vi "Making by Hot.vi"(0 "configuration file path":path caption="配置文件的路径", 1 "making by hot msic inf":T1) -> ()   [LabVIEW 2014]
uses:
  Ctl.xio/Making by Hot msic ctl.ctl
  SubVIS.xio/DataSocket/DataSocket_Tags.ctl
  Ctl.xio/part type.ctl
  SubVIS.xio/Creat Write List VI's/DefCtrl/Station.ctl
  <vilib>/Utility/file.llb/Read From Spreadsheet File (string).vi
panel:
  in  "SQL information":string
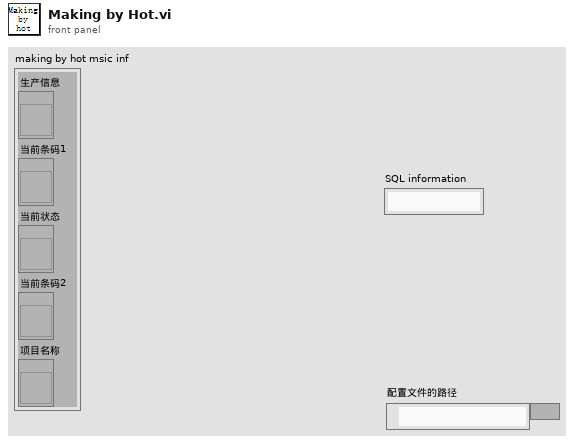
[diagram p1: front panel]
types:
  T1 = cluster{"生产信息":refnum<vi>, "当前条码1":refnum<vi>, "当前状态":refnum<vi>, "当前条码2":refnum<vi>, "项目名称":refnum<vi>}
  T2 = typedef "Station.ctl" = enum16{"粗切工位", "热处理工位", "精切工位", "PDF焊接工位", "打凹点预载力工位", "收卷工位", "EOL工位"}
  T3 = typedef "Making by Hot msic ctl.ctl" = cluster{"configuration file path":path, "DsOut":T4[], "BarCode1":string, "Hopper car information":cluster{"Hopper car code":string, "Hopper car No":string, "plate No":string}, "pallet.produced number":i32, "SQL information":string, "Database":string[], "Serial number":i32, "database path":path, "making by hot msic inf":cluster{"生产信息":refnum<vi>, "当前条码1":refnum<vi>, "当前状态":refnum<vi>, "当前条码2":refnum<vi>, "项目名称":refnum<vi>}, "scnner1 connect id":refnum<k5>, "scnner2 connect id":refnum<k5>, "scanner1 IP":string, "scanner2 IP":string, "BarCode2":string, "Heating process parameters":cluster{"heating start":string, "heating finish":string, "Heating time use":u32}, "part type":T5}
  T4 = typedef "DataSocket_Tags.ctl" = cluster{"Ds ID":refnum<k13>, "Tag":string}
  T5 = typedef "part type.ctl" = cluster{"项目号":string, "物料代码":string, "零件号":string, "供应商编码":string, "产线编码":string, "客户代码":string, "颜色代码":string, "托盘上限":i32, "加热温度":string, "加热时长":string, "EOL Stations":string}
  T6 = cluster{"Hopper car code":string, "Hopper car No":string, "plate No":string}
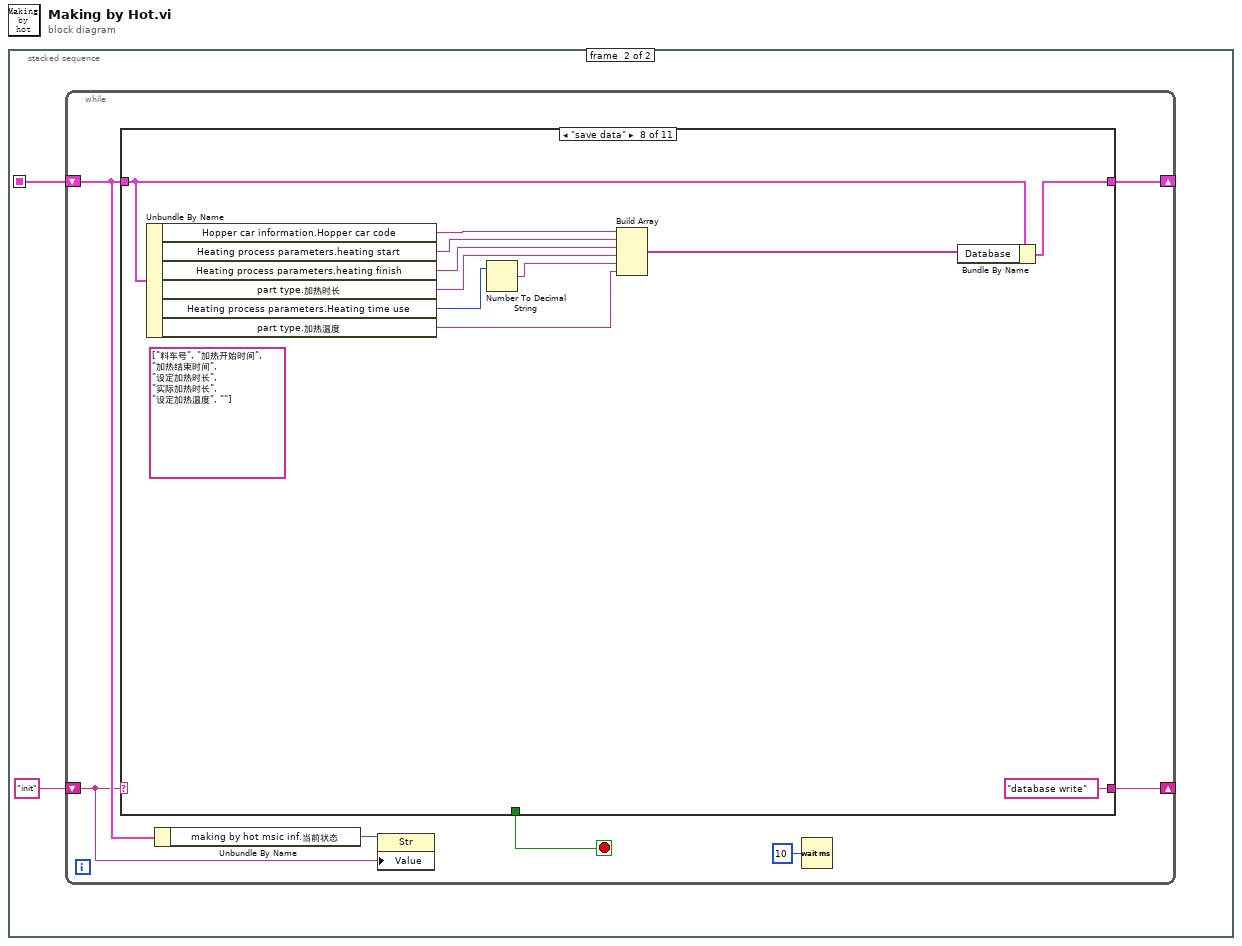
[diagram p0: block diagram]
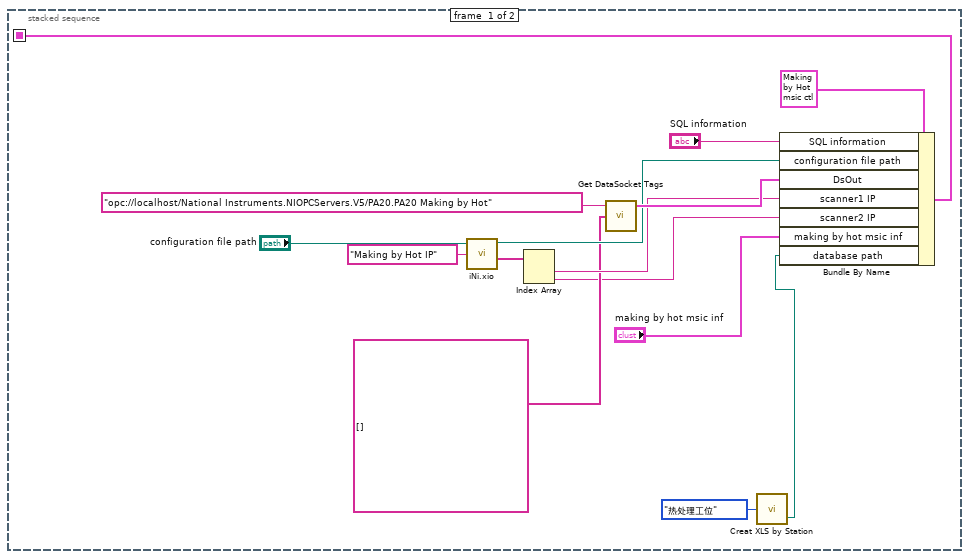
[diagram p2: hidden frame]
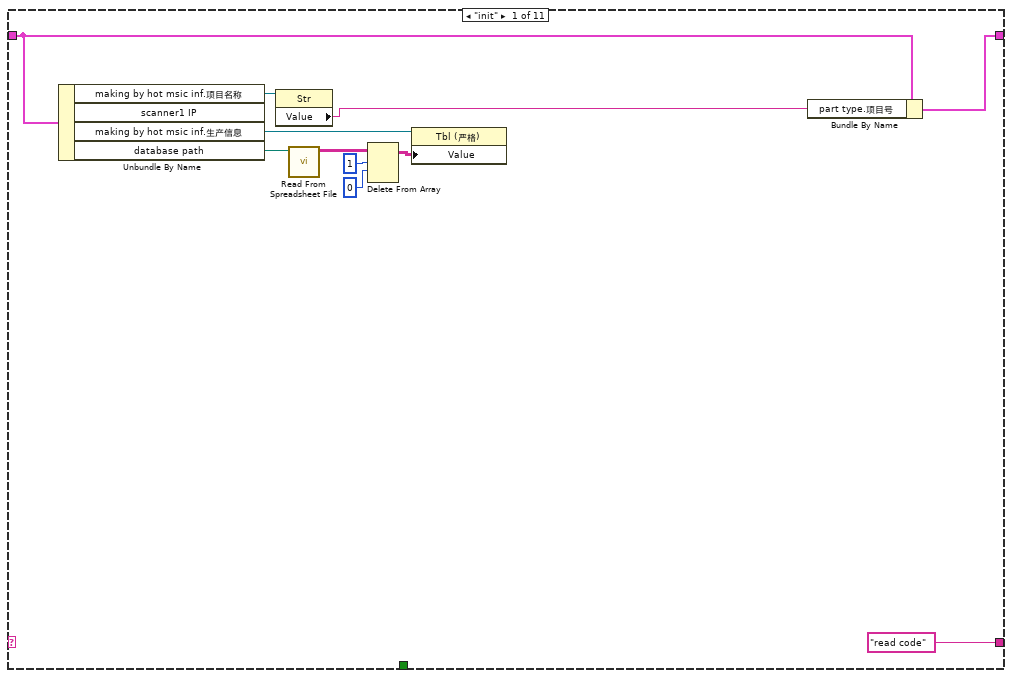
[diagram p3: hidden frame]
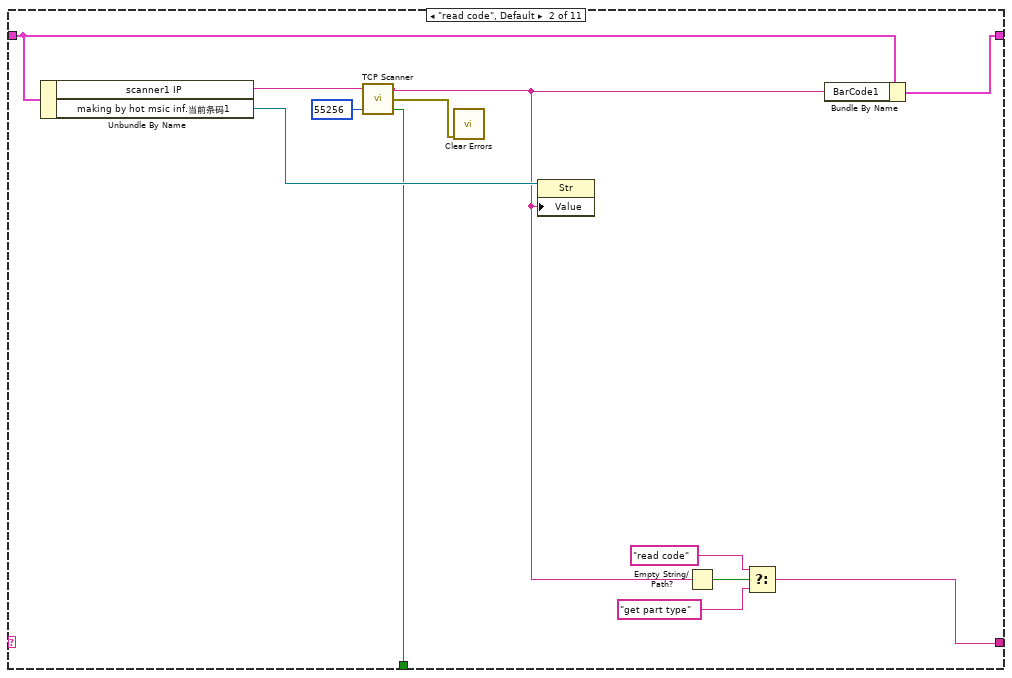
[diagram p4: hidden frame]
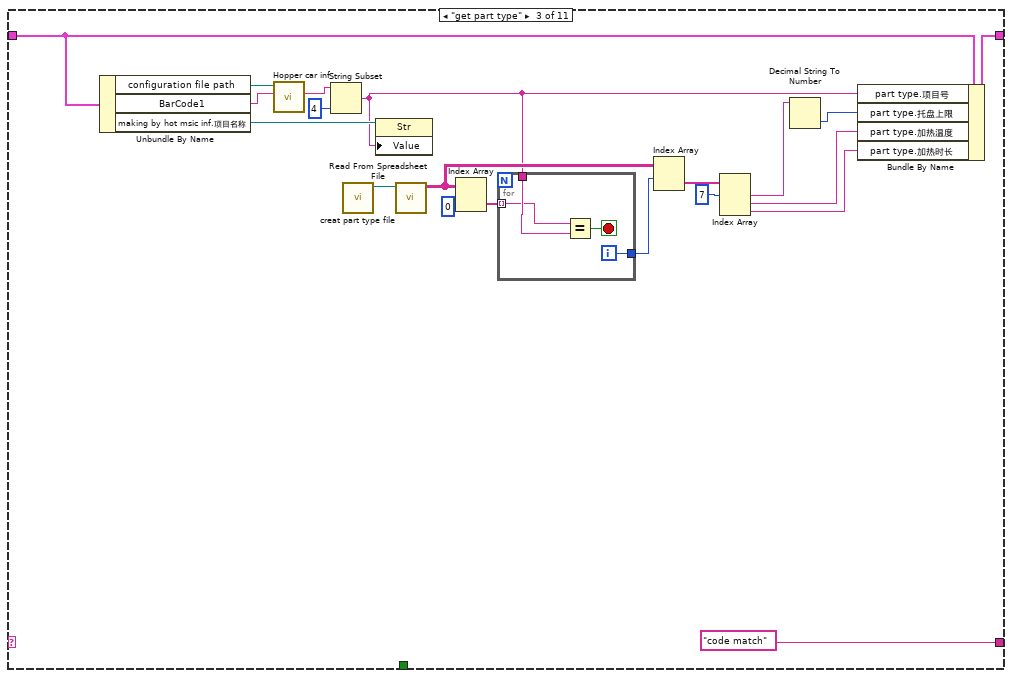
[diagram p5: hidden frame]
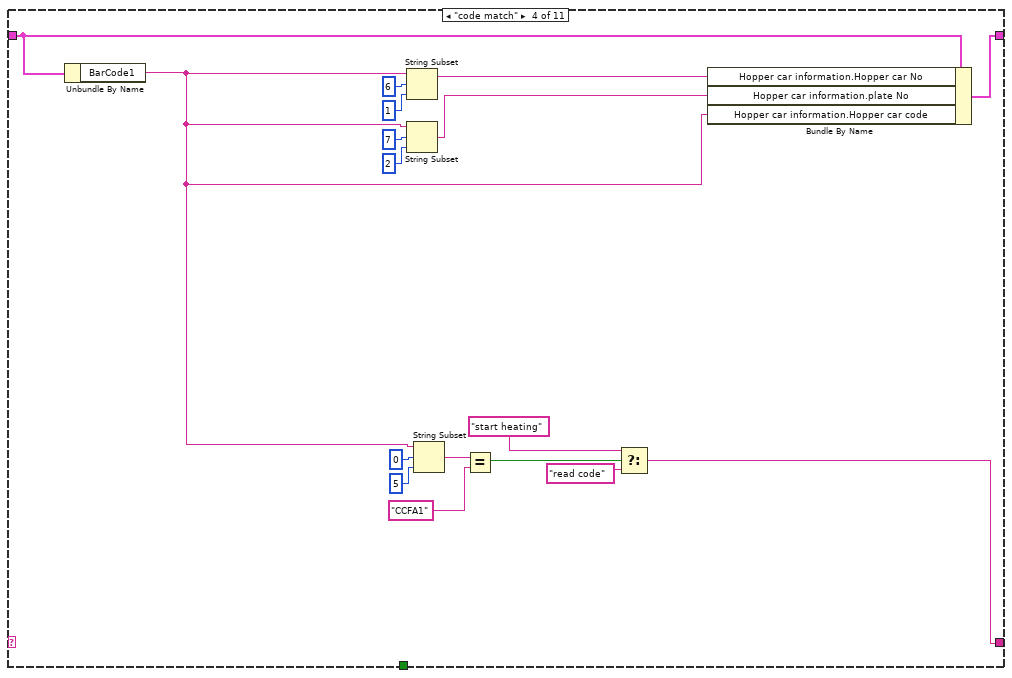
[diagram p6: hidden frame]
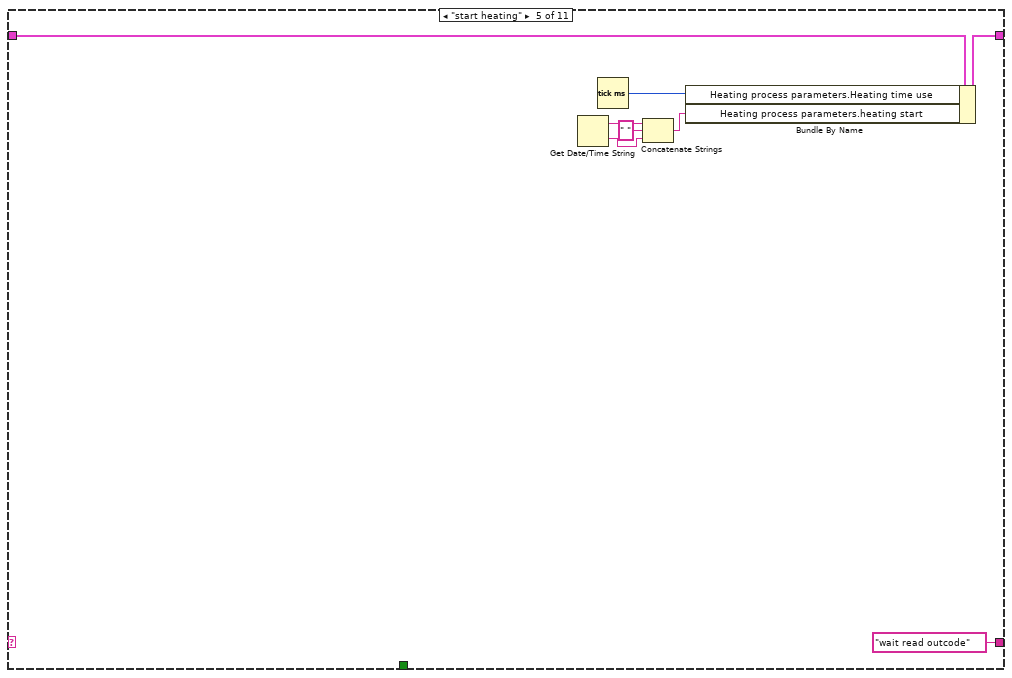
[diagram p7: hidden frame]
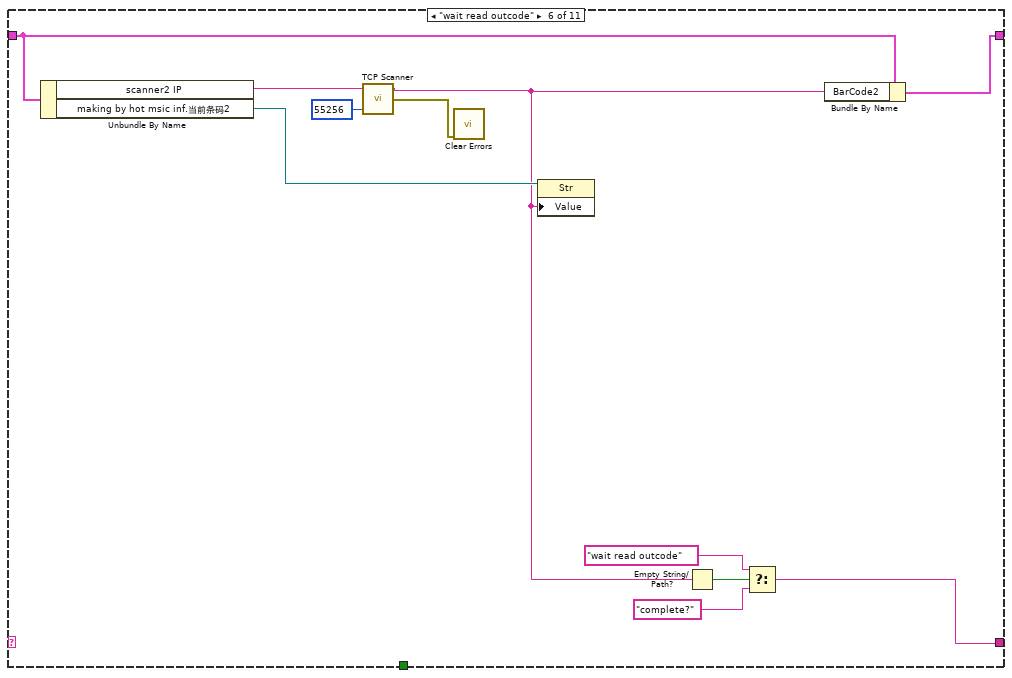
[diagram p8: hidden frame]
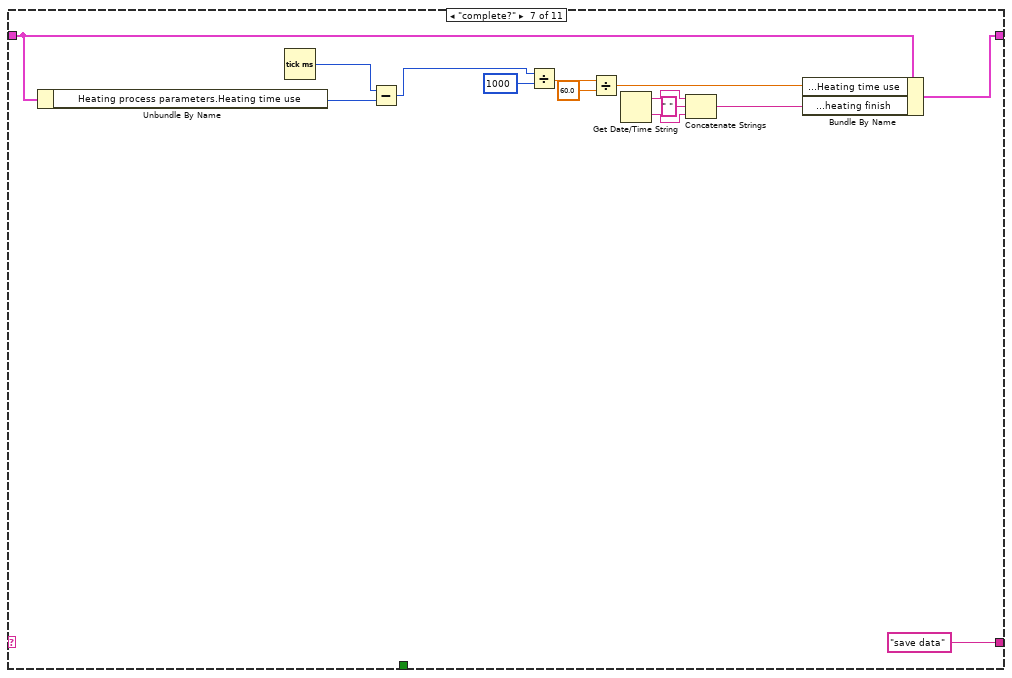
[diagram p9: hidden frame]
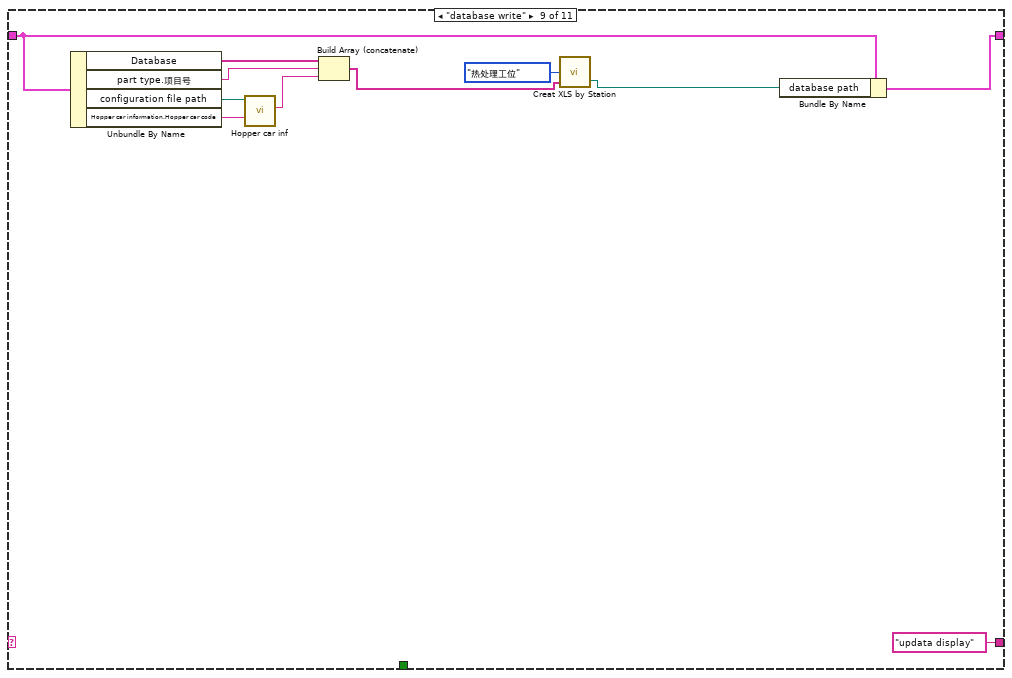
[diagram p10: hidden frame]
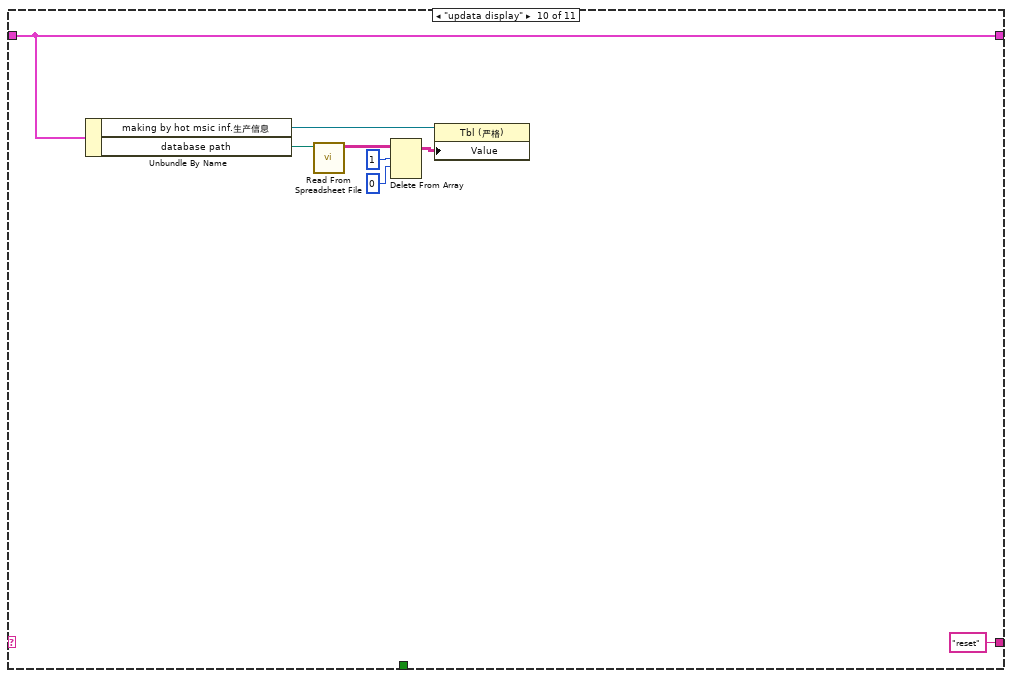
[diagram p11: hidden frame]
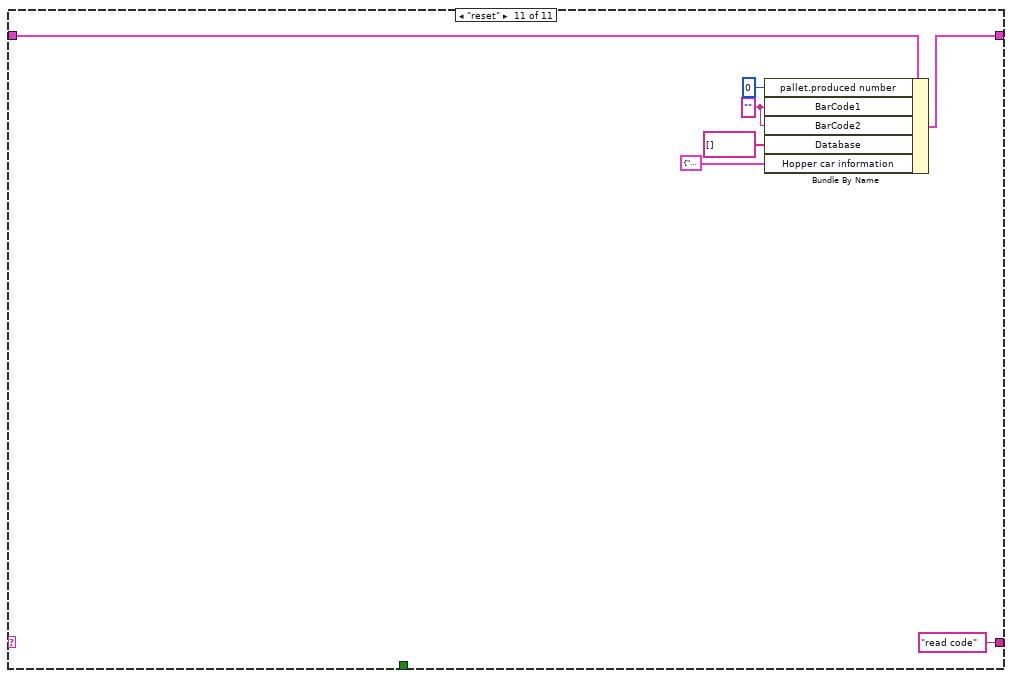
[diagram p12: hidden frame]
diagram:
  n1 = stacked-sequence {
    seq-local: [w3 _] -> [_ w16]
    frame #0 {
      n2 = call "iNi.xio.vi"("configuration file path"="configuration file path", "Sections"="Making by Hot IP") -> ("configuration file path"=w14:path, "Values"=w12:string[])  [unwired: 1 in, 3 out]
      n3 = Index Array(array=w12) -> (element #1=w11:string, element #2=w5:string)  [unwired: 2 in]
      n4 = call "Get DataSocket Tags.vi"("All Tags"=string[] [], "URL"="opc://localhost/National Instruments.NIOPCServers.V5/PA20.PA20 Making by Hot") -> ("DsOut"=w15:T4[])  [unwired: 3 in]
      n5 = call "Creat XLS by Station.vi"("staiton"=Station."热处理工位") -> ("new file path (Not A Path if cancelled)"=w1:path)  [unwired: 5 in]
      n6 = Bundle By Name(cluster=T3 {"configuration file path"=path "", "DsOut"=[], "BarCode1"="", "Hopper car information"={"Hopper car code"="", "Hopper car No"="", "plate No"=""}, "pallet.produced number"=0, "SQL information"="", "Database"=[], "Serial number"=0, "database path"=path "", "making by hot msic inf"={"生产信息"=refnum, "当前条码1"=refnum, "当前状态"=refnum, "当前条码2"=refnum, "项目名称"=refnum}, "scnner1 connect id"=refnum, "scnner2 connect id"=refnum, "scanner1 IP"="", "scanner2 IP"="", "BarCode2"="", "Heating process parameters"={"heating start"="", "heating finish"="", "Heating time use"=0}, "part type"={"项目号"="", "物料代码"="", "零件号"="", "供应商编码"="", "产线编码"="", "客户代码"="", "颜色代码"="", "托盘上限"=0, "加热温度"="", "加热时长"="", "EOL Stations"=""}} ("Making by Hot msic ctl"), "SQL information"="SQL information", "configuration file path"=w14, "DsOut"=w15, "scanner1 IP"=w11, "scanner2 IP"=w5, "making by hot msic inf"="making by hot msic inf", "database path"=w1) -> (w3:T3)
    }
    frame #1 {
      n7 = while {
        shift-right: [w24] -> _
        shift-left: w16 -> [w20]
        shift-right: [w23] -> _
        shift-left: "init" ("event") -> [w19]
        stop <- w18 stop-if-true
        n8 = case shown="\"save data\"" w19 {
          tunnel: w20 -> [w33 w45 w52 w73 w94 w105 w119 w131 w141 w148 w155]
          tunnel: [w35 w47 w67 w82 w96 w107 w114 w122 w142 w148 w157] -> w24
          tunnel: ["read code" w41 "code match" w80 "wait read outcode" ("event") w101 "save data" ("event") "database write" ("f") "updata display" ("f") "reset" ("f") "read code" ("f")] -> w23
          tunnel: [_ w36 _ _ _ _ _ _ _ _ _] -> w18
          frame "init" {
            n9 = Unbundle By Name(w33) -> ("making by hot msic inf.项目名称"=w32:refnum<vi>, "making by hot msic inf.生产信息"=w34:refnum<vi>, "database path"=w29:path)  [unwired: 1 out]
            n10 = property class="Str"(reference=w32) -> ("Value"=w31:string)  [unwired: 1 in, 2 out]
            n11 = call-poly <vilib>:"Read From Spreadsheet File.vi"("file path (dialog if empty)"=w29) -> ("all rows"=w26:string[][])  [unwired: 6 in, 4 out]
            n12 = Delete From Array(array=w26, length=1 ("长度"), index (row)=0 ("索引 (行)")) -> (array with subset deleted=w25:string[][])  [unwired: 1 in, 1 out]
            n13 = property class="Tbl (严格)"(reference=w34, "Value"=w25) -> ()  [unwired: 1 in, 2 out]
            n14 = Bundle By Name(cluster=w33, "part type.项目号"=w31) -> (w35:T3)
          }
          frame "read code", Default {
            n15 = Unbundle By Name(w45) -> ("scanner1 IP"=w39:string, "making by hot msic inf.当前条码1"=w46:refnum<vi>)
            n16 = call "TCP Scanner.vi"("Port（4001）"=u16 55256 ("远程端口或服务名称"), "ip"=w39) -> ("status"=w36:bool, "错误输出"=w37:errorcluster, "Barcode"=w38:string)  [unwired: 1 in]
            n17 = call <vilib>:"Clear Errors.vi"("error in (no error)"=w37) -> ()  [unwired: 5 in, 2 out]
            n18 = property class="Str"(reference=w46, "Value"=w38) -> ()  [unwired: 1 in, 2 out]
            n19 = Empty String/Path?(string/path=w38) -> (empty?=w44:bool)
            n20 = Select(t="read code" ("f"), s=w44, f="get part type") -> (s? t:f=w41:string)
            n21 = Bundle By Name(cluster=w45, "BarCode1"=w38) -> (w47:T3)
          }
          frame "get part type" {
            n22 = Unbundle By Name(w52) -> ("configuration file path"=w54:path, "BarCode1"=w53:string, "making by hot msic inf.项目名称"=w51:refnum<vi>)
            n23 = call "Hopper car inf.vi"("key"=w53, "path in"=w54) -> ("value out"=w50:string)  [unwired: 8 in, 1 out]
            n24 = String Subset(string=w50, length (rest)=4 ("长度（剩余）")) -> (substring=w48:string)  [unwired: 1 in]
            n25 = call "creat part type file.vi"() -> ("new file path (Not A Path if cancelled)"=w56:path)  [unwired: 11 in]
            n26 = property class="Str"(reference=w51, "Value"=w48) -> ()  [unwired: 1 in, 2 out]
            n27 = call-poly <vilib>:"Read From Spreadsheet File.vi"("file path (dialog if empty)"=w56) -> ("all rows"=w63:string[][])  [unwired: 6 in, 4 out]
            n28 = Index Array(array=w63, index (col)=0 ("禁用的索引 (列)")) -> (element=w65:string[])  [unwired: 1 in]
            n29 = for {
              tunnel: w65 -> [w68] mode=indexing
              tunnel: [w70] -> w62
              tunnel: w48 -> [w69]
              i -> [w70]
              stop <- w71 stop-if-true
              n30 = Equal?(x=w68, y=w69) -> (x = y?=w71:bool)
            }
            n31 = Index Array(array=w63, index (row)=w62) -> (element=w61:string[])  [unwired: 1 in]
            n32 = Index Array(array=w61, index #1=7 ("索引")) -> (element #1=w60:string, element #2=w58:string, element #3=w57:string)  [unwired: 2 in]
            n33 = Decimal String To Number(string=w60) -> (number=w59:i32)  [unwired: 2 in, 1 out]
            n34 = Bundle By Name(cluster=w52, "part type.项目号"=w48, "part type.托盘上限"=w59, "part type.加热温度"=w58, "part type.加热时长"=w57) -> (w67:T3)
          }
          frame "code match" {
            n35 = Unbundle By Name(w73) -> ("BarCode1"=w72:string)
            n36 = String Subset(string=w72, offset (0)=6 ("偏移量(0)"), length (rest)=1 ("长度（剩余）")) -> (substring=w75:string)
            n37 = String Subset(string=w72, offset (0)=7 ("偏移量(0)"), length (rest)=2 ("长度（剩余）")) -> (substring=w76:string)
            n38 = String Subset(string=w72, offset (0)=0 ("偏移量(0)"), length (rest)=5 ("长度（剩余）")) -> (substring=w77:string)
            n39 = Equal?(x=w77, y="CCFA1") -> (x = y?=w81:bool)
            n40 = Select(t="start heating" ("event"), s=w81, f="read code" ("event")) -> (s? t:f=w80:string)
            n41 = Bundle By Name(cluster=w73, "Hopper car information.Hopper car No"=w75, "Hopper car information.plate No"=w76, "Hopper car information.Hopper car code"=w72) -> (w82:T3)
          }
          frame "start heating" {
            n42 = Get Date/Time String() -> (date string=w92:string, time string=w90:string)  [unwired: 3 in]
            n43 = Tick Count (ms)() -> (millisecond timer value=w93:u32)
            n44 = Concatenate Strings(w92, " " ("字符串"), w90) -> (w89:string)
            n45 = Bundle By Name(cluster=w94, "Heating process parameters.Heating time use"=w93, "Heating process parameters.heating start"=w89) -> (w96:T3)
          }
          frame "wait read outcode" {
            n46 = Unbundle By Name(w105) -> ("scanner2 IP"=w99:string, "making by hot msic inf.当前条码2"=w106:refnum<vi>)
            n47 = call "TCP Scanner.vi"("Port（4001）"=u16 55256 ("远程端口或服务名称"), "ip"=w99) -> ("错误输出"=w97:errorcluster, "Barcode"=w98:string)  [unwired: 1 in, 1 out]
            n48 = call <vilib>:"Clear Errors.vi"("error in (no error)"=w97) -> ()  [unwired: 5 in, 2 out]
            n49 = property class="Str"(reference=w106, "Value"=w98) -> ()  [unwired: 1 in, 2 out]
            n50 = Empty String/Path?(string/path=w98) -> (empty?=w104:bool)
            n51 = Select(t="wait read outcode" ("f"), s=w104, f="complete?") -> (s? t:f=w101:string)
            n52 = Bundle By Name(cluster=w105, "BarCode2"=w98) -> (w107:T3)
          }
          frame "complete?" {
            n53 = Unbundle By Name(w119) -> ("Heating process parameters.Heating time use"=w120:u32)
            n54 = Tick Count (ms)() -> (millisecond timer value=w121:u32)
            n55 = Subtract(x=w121, y=w120) -> (x-y=w113:u32)
            n56 = Divide(x=w113, y=u32 1000) -> (x/y=w110:dbl)
            n57 = Divide(x=w110, y=60.0) -> (x/y=w108:dbl)
            n58 = Get Date/Time String() -> (date string=w115:string, time string=w117:string)  [unwired: 3 in]
            n59 = Concatenate Strings(w115, " " ("字符串"), w117) -> (w116:string)
            n60 = Bundle By Name(cluster=w119, "Heating process parameters.Heating time use"=w108, "Heating process parameters.heating finish"=w116) -> (w114:T3)
          }
          frame "save data" {
            (unwired) string[] ["料车号", "加热开始时间", "加热结束时间", "设定加热时长", "实际加热时长", "设定加热温度", ""] ("Header")
            n61 = Unbundle By Name(w131) -> ("Hopper car information.Hopper car code"=w130:string, "Heating process parameters.heating start"=w129:string, "Heating process parameters.heating finish"=w128:string, "part type.加热时长"=w127:string, "Heating process parameters.Heating time use"=w126:u32, "part type.加热温度"=w124:string)
            n62 = Number To Decimal String(number=w126) -> (decimal integer string=w125:string)  [unwired: 1 in]
            n63 = Build Array(w130, w129, w128, w127, w125, w124) -> (w123:string[])
            n64 = Bundle By Name(cluster=w131, "Database"=w123) -> (w122:T3)
          }
          frame "database write" {
            n65 = Unbundle By Name(w141) -> ("Database"=w140:string[], "part type.项目号"=w136:string, "configuration file path"=w139:path, "Hopper car information.Hopper car code"=w138:string)
            n66 = call "Hopper car inf.vi"("key"=w138, "path in"=w139) -> ("value out"=w137:string)  [unwired: 8 in, 1 out]
            n67 = Build Array (concatenate)(w140, w136, w137) -> (w133:string[])
            n68 = call "Creat XLS by Station.vi"("staiton"=Station."热处理工位", "data in"=w133) -> ("new file path (Not A Path if cancelled)"=w134:path)  [unwired: 4 in]
            n69 = Bundle By Name(cluster=w141, "database path"=w134) -> (w142:T3)
          }
          frame "updata display" {
            n70 = Unbundle By Name(w148) -> ("making by hot msic inf.生产信息"=w150:refnum<vi>, "database path"=w149:path)
            n71 = call-poly <vilib>:"Read From Spreadsheet File.vi"("file path (dialog if empty)"=w149) -> ("all rows"=w147:string[][])  [unwired: 6 in, 4 out]
            n72 = Delete From Array(array=w147, length=1 ("长度"), index (row)=0 ("索引 (行)")) -> (array with subset deleted=w144:string[][])  [unwired: 1 in, 1 out]
            n73 = property class="Tbl (严格)"(reference=w150, "Value"=w144) -> ()  [unwired: 1 in, 2 out]
          }
          frame "reset" {
            w154 = "" ("BarCode")
            n74 = Bundle By Name(cluster=w155, "pallet.produced number"=0, "BarCode1"=w154, "BarCode2"=w154, "Database"=string[] [], "Hopper car information"=T6 {"Hopper car code"="", "Hopper car No"="", "plate No"=""}) -> (w157:T3)
          }
        }
        n75 = Unbundle By Name(w20) -> ("making by hot msic inf.当前状态"=w21:refnum<vi>)
        n76 = property class="Str"(reference=w21, "Value"=w19) -> ()  [unwired: 1 in, 2 out]
        n77 = Wait (ms)(milliseconds to wait=u32 10 ("等待时间（毫秒）")) -> ()  [unwired: 1 out]
      }
    }
  }
